vi "RSNRPZ Get S-Parameter Device.vi"(8 "error in (no error)":errorcluster, 10 "Channel (1)":i32=1, 11 "VISA session":refnum<visa-resource-name> caption="VISA resource name") -> (0 "error out":errorcluster, 2 "S-Parameter":i32, 3 "dup VISA session":refnum<visa-resource-name> caption="VISA resource name")   [LabVIEW 2010]
doc: "This VI gets selected data set for S-parameter correction. \n\nNote(s):\n\n(1) This VI is available only on NRP-Z81.\n\nRemote-control command(s):\nSENS:CORR:SPD:SEL?"
uses:
  rsnrpz_32.dll
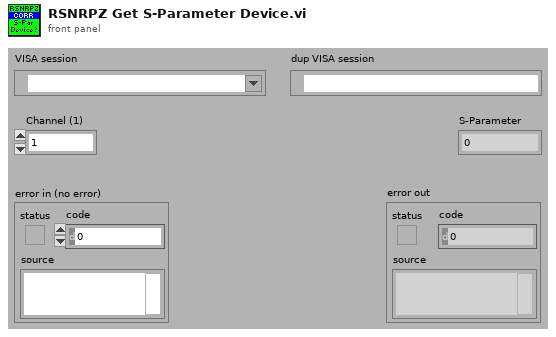
[diagram p1: front panel]
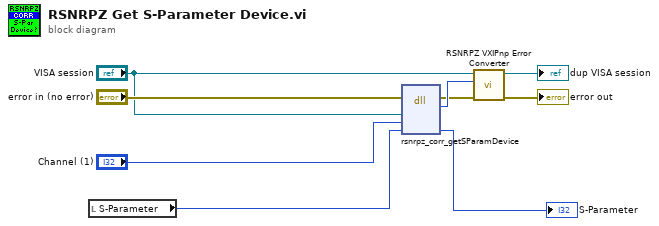
[diagram p0: block diagram]
diagram:
  n1 = local read "S-Parameter"() -> (w7:i32)
  n2 = dll-call lib="rsnrpz_32.dll" fn="rsnrpz_corr_getSParamDevice"(error in="error in (no error)", "Instrument Handle"="VISA session", "Channel"="Channel (1)", "S-Parameter"=w7) -> (error out=w5:errorcluster, "Status"=w9:i32, "S-Parameter"=→"S-Parameter":i32)  [unwired: 4 in, 1 out]
  n3 = call <instrlib>:"RSNRPZ VXIPnp Error Converter.vi"("error in"=w5, "VXIPnp error code"=w9, "VISA session"="VISA session") -> ("error out"=→"error out":errorcluster, "dup VISA session"=→"dup VISA session":refnum<visa-resource-name>)  [unwired: 7 in]
